vi "Mapping Merge Live Data.vi"(0 "New Spectrum":T2, 1 "Target Position":T1={"Drive X Set"=10.0, "Drive Y Set"=10.0, "Drive Z Set"=10.0} {"Drive X Set" min=10.0 max=160.0 step=0.1 format="%.1f"; "Drive Z Set" min=10.0 max=160.0 step=0.1 format="%.1f"; "Drive Y Set" min=10.0 max=160.0 step=0.1 format="%.1f"}, 5 "X in (1D)":dbl[](array[numeric]), 7 "Y in (1D)":dbl[](array[numeric]), 9 "L in (2D)":dbl[][](array[numeric]), 11 "I in (2D)":dbl[][](array[numeric])) -> (4 "Live Data":dbl[][](array[numeric]), 6 "X out (1D)":dbl[](array[numeric]), 8 "Y out (1D)":dbl[](array[numeric]), 10 "L out (2D)":dbl[][](array[numeric]), 15 "I out (2D)":dbl[][](array[numeric]))   [LabVIEW 2010]
uses:
  ESA-C/TypeDefs/ESA-C Set Positions.ctl
panel:
  # "Target positions to provide equidistance for Raman Tool Set"
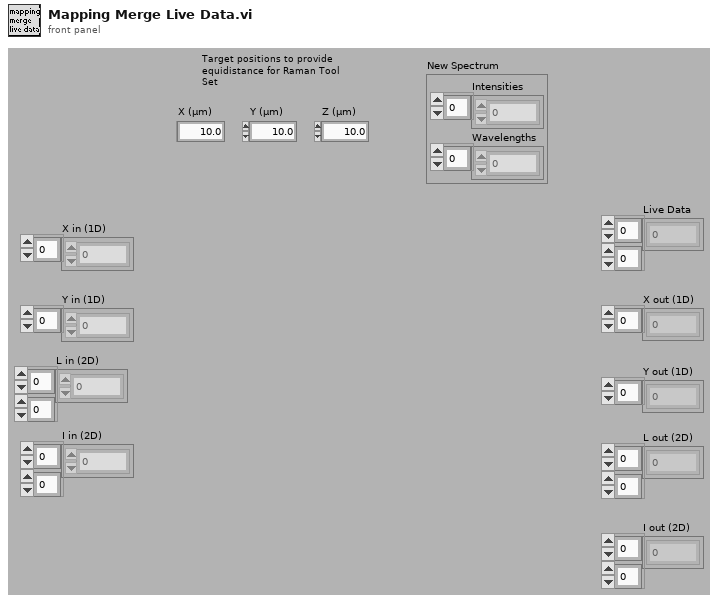
[diagram p1: front panel]
types:
  T1 = typedef "ESA-C Set Positions.ctl" = cluster{"Drive X Set":dbl, "Drive Y Set":dbl, "Drive Z Set":dbl}
  T2 = cluster{"Intensities":dbl[], "Wavelengths":dbl[]}
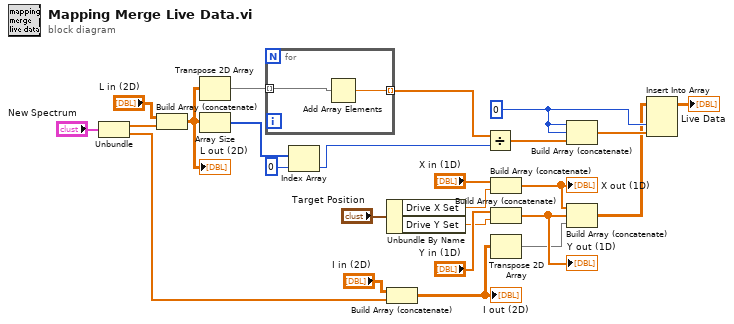
[diagram p0: block diagram]
diagram:
  w7 = 0
  n1 = Unbundle("New Spectrum") -> ("Intensities"=w25:dbl[], "Wavelengths"=w24:dbl[])
  n2 = Build Array (concatenate)("L in (2D)", w25) -> (w20:dbl[][])
  "L out (2D)" <- w20
  n3 = Transpose 2D Array(2D array=w20) -> (transposed array=w21:dbl[][])
  n4 = Array Size(array=w20) -> (size(s)=w13:i32[])
  n5 = for {
    tunnel: [w27] -> w11 mode=indexing
    tunnel: w21 -> [w26] mode=indexing
    n6 = Add Array Elements(numeric array=w26) -> (sum=w27:dbl)
  }
  n7 = Index Array(array=w13, index=0 ("Index")) -> (element=w15:i32)
  n8 = Unbundle By Name("Target Position") -> ("Drive X Set"=w5:dbl, "Drive Y Set"=w6:dbl)
  n9 = Build Array (concatenate)("I in (2D)", w24) -> (w19:dbl[][])
  "I out (2D)" <- w19
  n10 = Divide(x=w11, y=w15) -> (x/y=w12:dbl[])
  n11 = Build Array (concatenate)("X in (1D)", w5) -> (w17:dbl[])
  "X out (1D)" <- w17
  n12 = Build Array (concatenate)("Y in (1D)", w6) -> (w18:dbl[])
  "Y out (1D)" <- w18
  n13 = Transpose 2D Array(2D array=w19) -> (transposed array=w4:dbl[][])
  n14 = Build Array (concatenate)(w7, w7, w12) -> (w3:dbl[])
  n15 = Build Array (concatenate)(w17, w18, w4) -> (w2:dbl[][])
  n16 = Insert Into Array(array=w2, index (col)=w7, new element=w3) -> (→"Live Data":dbl[][])  [unwired: 1 in]
